vi "auto avance ralentir.vi"(8 "Temps reculer":dbl, 9 "vitesse gauche":dbl, 10 "temps avancer":dbl, 11 "temps de changement de direction":dbl) -> ()   [LabVIEW 2015]
uses:
  <vilib>/Rock Robotics/WPI/Solenoid/WPI_SolenoidValue.ctl
  <vilib>/Rock Robotics/WPI/Solenoid/WPI_SolenoidSetEnum.vi
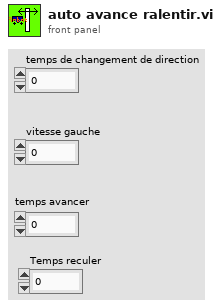
[diagram p1: front panel]
types:
  T1 = typedef "WPI_SolenoidValue.ctl" = enum16{"Off", "On", "Forward", "Reverse"}
  T2 = typedef "WPI_ServoDeviceRef.ctl" = cluster{"DeviceStatus":errorcluster, "PWM Channel":T3, "DeadBand":T4}
  T3 = typedef "FPGA_DIOPWMChannel.ctl" = enum8{"PWM 0", "PWM 1", "PWM 2", "PWM 3", "PWM 4", "PWM 5", "PWM 6", "PWM 7", "PWM 8", "PWM 9", "PWM MXP 0", "PWM MXP 1", "PWM MXP 2", "PWM MXP 3", "PWM MXP 4", "PWM MXP 5", "PWM MXP 6", "PWM MXP 7", "PWM MXP 8", "PWM MXP 9", "Invalid"}
  T4 = typedef "WPI_PWMDeadband.ctl" = cluster{"Name":string, "maxPositivePwm":i32, "minPositivePwm":i32, "centerPwm":i32, "maxNegativePwm":i32, "minNegativePwm":i32, "angularRange":u16}
  T5 = typedef "WPI_SolenoidDevRef.ctl" = cluster{"DevStatus":errorcluster, "Pneumatics Control Module":u8, "Forward Solenoid Channel":T6, "Reverse Solenoid Channel":T6}
  T6 = typedef "WPI_SolenoidChannel.ctl" = enum8{"Solenoid 0", "Solenoid 1", "Solenoid 2", "Solenoid 3", "Solenoid 4", "Solenoid 5", "Solenoid 6", "Solenoid 7", "Invalid"}
  T7 = typedef "WPI_EncoderDevRef.ctl" = cluster{"DevStatus":errorcluster, "EncoderIndex":T8, "CounterIndex":T9, "DistancePerCount":dbl, "Decoding Type":T10}
  T8 = typedef "FPGA_EncoderIdx.ctl" = enum8{"Enc 0", "Enc 1", "Enc 2", "Enc 3", "Enc 4", "Enc 5", "Enc 6", "Enc 7", "Invalid"}
  T9 = typedef "FPGA_CounterCtrSystemIndex.ctl" = enum8{"Ctr 0", "Ctr 1", "Ctr 2", "Ctr 3", "Ctr 4", "Ctr 5", "Ctr 6", "Ctr 7", "Invalid"}
  T10 = typedef "WPI_EncoderType.ctl" = enum16{"1x", "2x", "4x"}
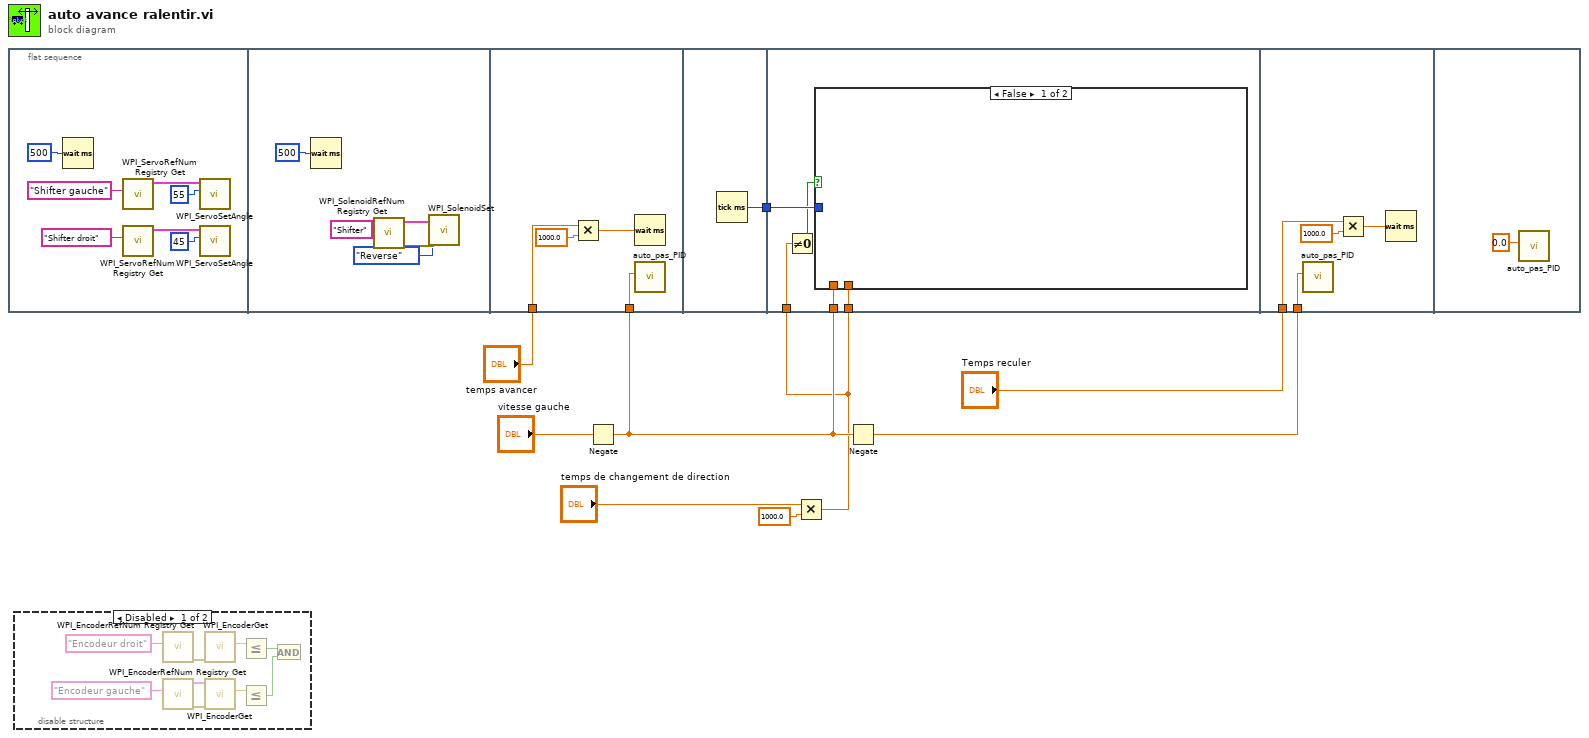
[diagram p0: block diagram]
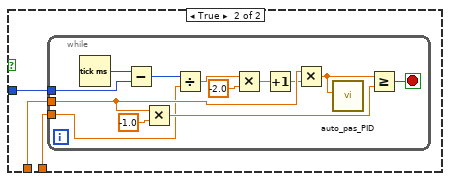
[diagram p2: hidden frame]
diagram:
  n1 = flat-sequence {
    tunnel: w5 -> [w25]
    tunnel: "temps avancer" -> [w23]
    tunnel: [w26] -> w9
    tunnel: w9 -> [w31]
    tunnel: w5 -> [w30]
    tunnel: w1 -> [w29]
    tunnel: w1 -> [w27]
    tunnel: w4 -> [w51]
    tunnel: "Temps reculer" -> [w48]
    frame #0 {
      n2 = Wait (ms)(milliseconds to wait=u32 500) -> ()  [unwired: 1 out]
      n3 = call <vilib>:"WPI_ServoRefNum Registry Get.vi"("refnum name"="Shifter gauche") -> ("ServoDeviceRef"=w15:T2)  [unwired: 9 in, 1 out]
      n4 = call <vilib>:"WPI_ServoRefNum Registry Get.vi"("refnum name"="Shifter droit") -> ("ServoDeviceRef"=w16:T2)  [unwired: 9 in, 1 out]
      n5 = call <vilib>:"WPI_ServoSetAngle.vi"("Angle"=55, "ServoDeviceRef"=w15) -> ()  [unwired: 8 in, 2 out]
      n6 = call <vilib>:"WPI_ServoSetAngle.vi"("Angle"=45, "ServoDeviceRef"=w16) -> ()  [unwired: 8 in, 2 out]
    }
    frame #1 {
      n7 = Wait (ms)(milliseconds to wait=u32 500) -> ()  [unwired: 1 out]
      n8 = call <vilib>:"WPI_SolenoidRefNum Registry Get.vi"("refnum name"="Shifter") -> ("error out"=w19:errorcluster, "SolenoidDevRef"=w18:T5)  [unwired: 9 in]
      n9 = call-poly <vilib>:"WPI_SolenoidSet.vi"("error in (no error)"=w19, "Value"=WPI_SolenoidValue."Reverse", "SolenoidDevRef"=w18) -> ()  [unwired: 7 in, 2 out]
    }
    frame #2 {
      n10 = Multiply(x=w23, y=1000.0) -> (x*y=w22:dbl)
      n11 = Wait (ms)(milliseconds to wait=w22) -> ()  [unwired: 1 out]
      n12 = call "auto_pas_PID.vi"("vitesse voulu"=w25) -> ()  [unwired: 11 in]
    }
    frame #3 {
      n13 = Tick Count (ms)() -> (millisecond timer value=w26:u32)
    }
    frame #4 {
      n14 = Not Equal To 0?(x=w27) -> (x != 0?=w28:bool)
      n15 = case shown="False" w28 {
        tunnel: w31 -> [_ w34]
        tunnel: w30 -> [_ w33]
        tunnel: w29 -> [_ w32]
        frame False {
        }
        frame True {
          n16 = while {
            tunnel: w34 -> [w38]
            tunnel: w33 -> [w46]
            tunnel: w32 -> [w44]
            stop <- w35 stop-if-true
            n17 = Tick Count (ms)() -> (millisecond timer value=w37:u32)
            n18 = Subtract(x=w37, y=w38) -> (x-y=w43:u32)
            n19 = Multiply(x=w46, y=-1.0) -> (x*y=w45:dbl)
            n20 = Divide(x=w43, y=w44) -> (x/y=w41:dbl)
            n21 = Multiply(x=w41, y=-2.0) -> (x*y=w40:dbl)
            n22 = Increment(x=w40) -> (x+1=w39:dbl)
            n23 = Multiply(x=w46, y=w39) -> (x*y=w36:dbl)
            n24 = call "auto_pas_PID.vi"("vitesse voulu"=w36) -> ()  [unwired: 11 in]
            n25 = Greater Or Equal?(x=w36, y=w45) -> (x >= y?=w35:bool)
          }
        }
      }
    }
    frame #5 {
      n26 = call "auto_pas_PID.vi"("vitesse voulu"=w51) -> ()  [unwired: 11 in]
      n27 = Multiply(x=w48, y=1000.0) -> (x*y=w50:dbl)
      n28 = Wait (ms)(milliseconds to wait=w50) -> ()  [unwired: 1 out]
    }
    frame #6 {
      n29 = call "auto_pas_PID.vi"("vitesse voulu"=0.0) -> ()  [unwired: 11 in]
    }
  }
  n30 = disable-structure shown="Disabled" {
    frame Disabled {
      n31 = call <vilib>:"WPI_EncoderRefNum Registry Get.vi"("refnum name"="Encodeur droit") -> ("error out"=w53:errorcluster)  [unwired: 9 in, 1 out]
      n32 = call <vilib>:"WPI_EncoderRefNum Registry Get.vi"("refnum name"="Encodeur gauche") -> ("error out"=w55:errorcluster, "EncoderDevRef"=w56:T7)  [unwired: 9 in]
      n33 = call <vilib>:"WPI_EncoderGet.vi"("error in (no error)"=w53) -> ("Distance"=w58:dbl)  [unwired: 5 in, 5 out]
      n34 = call <vilib>:"WPI_EncoderGet.vi"("error in (no error)"=w55, "EncoderDevRef"=w56) -> ("Distance"=w61:dbl)  [unwired: 4 in, 5 out]
      n35 = Less Or Equal?(x=w58) -> (x <= y?=w59:bool)  [unwired: 1 in]
      n36 = Less Or Equal?(x=w61) -> (x <= y?=w60:bool)  [unwired: 1 in]
      n37 = And(x=w59, y=w60) -> ()  [unwired: 1 out]
    }
    frame Enabled {
    }
  }
  n38 = Negate(x="vitesse gauche") -> (-x=w5:dbl)
  n39 = Multiply(x="temps de changement de direction", y=1000.0) -> (x*y=w1:dbl)
  n40 = Negate(x=w5) -> (-x=w4:dbl)
